vi "reset AO_DO_v3.vi"() -> ()   [LabVIEW 2015]
uses:
  <vilib>/DAQmx/write.llb/DAQmx Write (Analog 1D Wfm NChan NSamp).vi
  <vilib>/DAQmx/write.llb/DAQmx Write (Digital 1D Wfm NChan NSamp).vi
  waveforms/usedDOindepofwf.vi
  waveforms/usedAOindepofwf.vi
  Misc/add channel to active arrayv2.vi
  <vilib>/Waveform/DWDTOps.llb/DWDT Analog to Digital.vi
  <vilib>/Waveform/DWDTOps.llb/DWDT Uncompress Digital.vi
  <vilib>/DAQmx/miscellaneous.llb/DAQmx Fill In Error Info.vi
panel:
  out "number of samples written per channel":u32
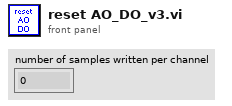
[diagram p1: front panel]
types:
  T1 = cluster{"VC":bool, "CC":bool, "CC_icg (pA/mv)":sgl, "VC_icg (mV/mV)":sgl, "OCG (mV/pA)":sgl, "OVG (mV/mV)":dbl, "Vhold (mV)":sgl, "holdon":bool}
  T2 = typedef "LVRectTypeDef.ctl" = cluster{"Left":i16, "Top":i16, "Right":i16, "Bottom":i16}
  T3 = cluster{"Xpixels":i32, "Vxminref":dbl, "Vxmaxref":dbl, "P":dbl, "Ypixels":i32, "Vyminref":dbl, "Vymaxref":dbl, "srate":sgl, "sAOxy":i32, "timeout":dbl, "type":string, "date":string, "time":string, "Colormap":u16, "Drawing Mode":u16, "Scanning Mode":u16, "square pixels":bool, "square matrix":bool, "Xpixels Img":i32, "Vx-min Img":dbl, "VX-max Img":dbl, "Ypixels Img":i32, "Vy-min Img":dbl, "Vy-max Img ":dbl, "Angle Img":dbl, "autoshutter":bool, "finite":bool, "cont":bool, "wavdet":bool, "measpoints":i32, "avpp":i32, "bufferAO":i32, "bufferAI":i32, "starttick":u32, "waveform":path, "Vx-ref":dbl, "Vy-ref":dbl, "refreshrate":dbl, "refreshbuffer":i32, "tt_cycles":i32, "motorref":refnum<k7>, "mirrorswitch":refnum<k7>, "sample mode":i32, "maxbufferAI":i32, "srateAODO":sgl, "bin":sgl, "Pel":sgl, "Angle draw":dbl, "srate Img":sgl, "ROIimg_plotbounds":T2, "auto OD":bool, "ODfilt":u16, "aAI":i32[], "aCI":i32[], "aAO":u32[], "aDO":u32[], "refwfsize":dbl, "Lifetime":bool, "Vz-Img":dbl, "Vz-ref":dbl, "Vz-reset":dbl, "AIoverride":bool}
  T4 = cluster{"AO":refnum<k21>[], "E_AO":errorcluster[]}
  T5 = cluster{"StageS":i32, "StageL":i32, "currmeas data dir":path, "image OD":u16, "contour OD":u16, "point OD":u16, "AOlines":tag[], "AIlines":tag[], "CI lines":tag[], "DO lines":tag[], "AO names":string[], "CI names":string[], "AI names":string[], "DO names":string[], "CIextensions":string[], "AIextensions":string[], "Voltage to Ygalvo":i32, "Voltage to Xgalvo":i32, "Voltage to patch":i32, "640 shutter":i32, "2P shutter":i32, "LT timestamp":u32, "Vp":i32, "Ip":i32, "camera trigger":i32, "master data dir":path, "voltage to Zpos":i32, "Vto2P":i32, "640 AO":i32, "488 AO":i32, "532 AO":i32, "640TTL":u32, "488TTL":u32, "532TTL":u32, "Device 1 sampleclock out":tag, "Device 1 Starttrigger out":tag, "Device 2 sampleclock in":tag, "Device 2 StartTrigger in ":tag, "2PODTTL":u32, "488 shutter":u32, "LCVR red":u32, "LCVR blue":u32}
  T6 = cluster{"presorted indices":i32[], "AOchans in this device":tag[], "usedAO sorted":i32[]}[]
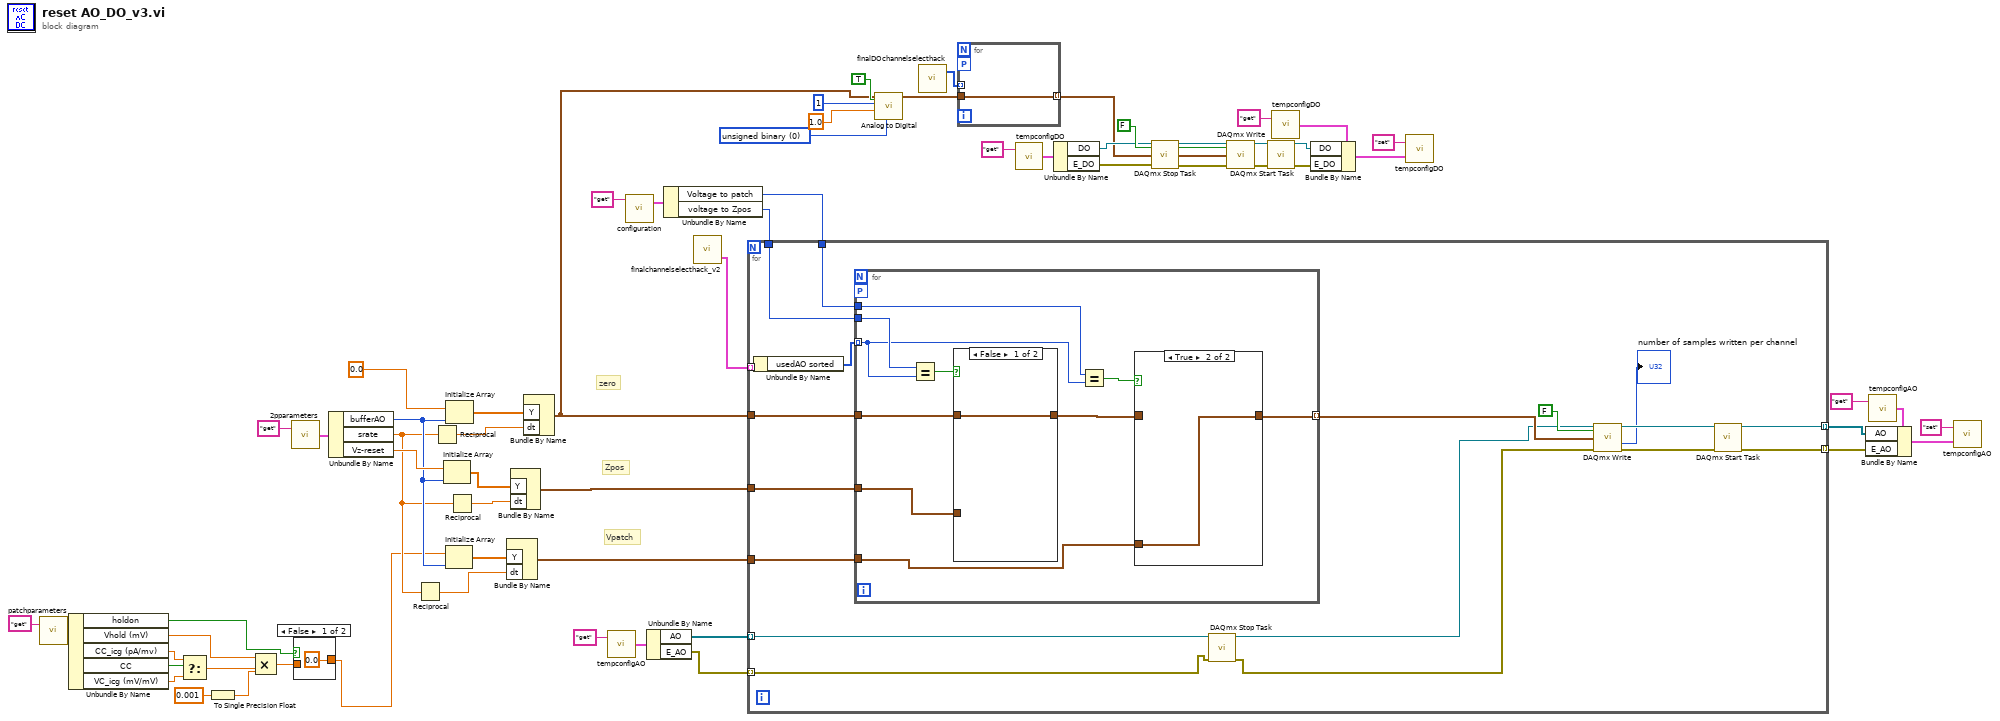
[diagram p0: block diagram]
diagram:
  w50 = u16 0 items=["unsigned binary", "offset binary", "2's complement"] ("data format (offset binary)")
  # "Vpatch"
  # "Zpos"
  # "zero"
  n1 = call "patchparameters.vi"("command"="get") -> ("Params out"=w10:T1)  [unwired: 1 in]
  n2 = Unbundle By Name(w10) -> ("holdon"=w11:bool, "Vhold (mV)"=w12:sgl, "CC_icg (pA/mv)"=w4:sgl, "CC"=w6:bool, "VC_icg (mV/mV)"=w5:sgl)
  n3 = Select(t=w4, s=w6, f=w5) -> (s? t:f=w3:sgl)
  n4 = To Single Precision Float(number=0.001 ("y")) -> (single precision float=w2:sgl)
  n5 = Compound Arithmetic op=MULTIPLY(w12, w3, w2) -> (w8:sgl)
  n6 = call "2pparameters.vi"("command"="get") -> ("params out"=w41:T3)  [unwired: 1 in]
  n7 = case shown="False" w11 {
    tunnel: w8 -> [_ w66]
    tunnel: [0.0 w66] -> w1
    frame False {
    }
    frame True {
    }
  }
  n8 = Unbundle By Name(w41) -> ("bufferAO"=w30:i32, "srate"=w29:sgl, "Vz-reset"=w35:dbl)
  n9 = Reciprocal(x=w29) -> (1/x=w39:sgl)
  n10 = Reciprocal(x=w29) -> (1/x=w46:sgl)
  n11 = Initialize Array(w35, w30) -> (w37:dbl[])
  n12 = Initialize Array(w1, w30) -> (w38:dbl[])
  n13 = Initialize Array(0.0 ("element"), w30) -> (w48:dbl[])
  n14 = Reciprocal(x=w29) -> (1/x=w36:sgl)
  n15 = Bundle By Name("Y"=w38, "dt"=w39) -> (w27:waveform(dbl))  [unwired: 1 in]
  n16 = Bundle By Name("Y"=w37, "dt"=w36) -> (w28:waveform(dbl))  [unwired: 1 in]
  n17 = Bundle By Name("Y"=w48, "dt"=w46) -> (w40:waveform(dbl))  [unwired: 1 in]
  n18 = call "tempconfigAO.vi"("command"="get") -> ("Temp Config out"=w22:T4)  [unwired: 1 in]
  n19 = call "configuration.vi"("command"="get") -> ("config out"=w33:T5)  [unwired: 2 in, 1 out]
  n20 = Unbundle By Name(w22) -> ("AO"=w20:refnum<k21>[], "E_AO"=w19:errorcluster[])
  n21 = Unbundle By Name(w33) -> ("Voltage to patch"=w32:i32, "voltage to Zpos"=w31:i32)
  n22 = call "finalchannelselecthack_v2.vi"() -> ("Device chans"=w23:T6)  [unwired: 1 in, 1 out]
  n23 = for {
    tunnel: [w69] -> w44 mode=indexing
    tunnel: w40 -> [w82]
    tunnel: w32 -> [w81]
    tunnel: w31 -> [w80]
    tunnel: w28 -> [w79]
    tunnel: w27 -> [w78]
    tunnel: [w67] -> w24 mode=indexing
    tunnel: w23 -> [w75] mode=indexing
    tunnel: w20 -> [w73] mode=indexing
    tunnel: w19 -> [w71] mode=indexing
    n24 = Unbundle By Name(w75) -> ("usedAO sorted"=w74:i32[])
    n25 = for {
      tunnel: w82 -> [w89]
      tunnel: w74 -> [w92] mode=indexing
      tunnel: w81 -> [w94]
      tunnel: w80 -> [w93]
      tunnel: [w87] -> w77 mode=indexing
      tunnel: w79 -> [w86]
      tunnel: w78 -> [w85]
      workers-P: _ -> [_]
      n26 = Equal?(x=w93, y=w92) -> (x = y?=w91:bool)
      n27 = case shown="False" w91 {
        tunnel: w89 -> [w97 _]
        tunnel: [w97 w98] -> w88
        tunnel: w86 -> [_ w98]
        frame False {
        }
        frame True {
        }
      }
      n28 = Equal?(x=w94, y=w92) -> (x = y?=w90:bool)
      n29 = case shown="True" w90 {
        tunnel: w88 -> [w95 _]
        tunnel: [w95 w96] -> w87
        tunnel: w85 -> [_ w96]
        frame False {
        }
        frame True {
        }
      }
    }
    n30 = call <vilib>:"DAQmx Stop Task.vi"("task/channels in"=w73, "error in"=w71) -> ("task out"=w72:refnum<k21>, "error out"=w70:errorcluster)  [unwired: 12 in]
    n31 = call-poly <vilib>:"DAQmx Write.vi"("task/channels in"=w72, "auto start"=FALSE, "data"=w77, "error in"=w70) -> ("task out"=w83:refnum<k21>, "number of samples written per channel"=→"number of samples written per channel":u32, "error out"=w68:errorcluster)  [unwired: 9 in]
    n32 = call <vilib>:"DAQmx Start Task.vi"("task/channels in"=w83, "error in"=w68) -> ("task out"=w69:refnum<k21>, "error out"=w67:errorcluster)  [unwired: 12 in]
  }
  n33 = call-poly <vilib>:"Analog to Digital.vi"("data format (offset binary)"=w50, "compress digital (T)"=TRUE, "full-scale range (pk-pk)"=1.0, "resolution (16 bit)"=1, "analog waveform"=w40) -> ("digital waveform"=w49:digitalwaveform)  [unwired: 3 in, 3 out]
  n34 = call "finalDOchannelselecthack.vi"() -> ("usedDO"=w26:u32[])  [unwired: 1 in, 1 out]
  n35 = for {
    tunnel: [w99] -> w25 mode=indexing
    tunnel: w49 -> [w99]
    tunnel: w26 -> [_] mode=indexing
    workers-P: _ -> [_]
  }
  n36 = call "tempconfigDO.vi"("command"="get") -> ("Temp Config out"=w55:cluster{"DO":refnum<k21>, "E_DO":errorcluster})  [unwired: 1 in]
  n37 = Unbundle By Name(w55) -> ("DO"=w54:refnum<k21>, "E_DO"=w15:errorcluster)
  n38 = call <vilib>:"DAQmx Stop Task.vi"("task/channels in"=w54, "error in"=w15) -> ("task out"=w16:refnum<k21>, "error out"=w14:errorcluster)  [unwired: 12 in]
  n39 = call-poly <vilib>:"DAQmx Write.vi"("task/channels in"=w16, "auto start"=FALSE, "data"=w25, "error in"=w14) -> ("task out"=w43:refnum<k21>, "error out"=w17:errorcluster)  [unwired: 9 in, 1 out]
  n40 = call <vilib>:"DAQmx Start Task.vi"("task/channels in"=w43, "error in"=w17) -> ("task out"=w18:refnum<k21>, "error out"=w13:errorcluster)  [unwired: 12 in]
  n41 = call "tempconfigDO.vi"("command"="get") -> ("Temp Config out"=w61:cluster{"DO":refnum<k21>, "E_DO":errorcluster})  [unwired: 1 in]
  n42 = Bundle By Name(cluster=w61, "DO"=w18, "E_DO"=w13) -> (w63:cluster{"DO":refnum<k21>, "E_DO":errorcluster})
  n43 = call "tempconfigDO.vi"("Temp Config in"=w63, "command"="set") -> ()  [unwired: 1 out]
  n44 = call "tempconfigAO.vi"("command"="get") -> ("Temp Config out"=w58:T4)  [unwired: 1 in]
  n45 = Bundle By Name(cluster=w58, "AO"=w44, "E_AO"=w24) -> (w59:T4)
  n46 = call "tempconfigAO.vi"("Temp Config in"=w59, "command"="set") -> ()  [unwired: 1 out]
